vi "Build Tx-UDP Cluster.vi"(0 "section ref in":T8=18446744073709551615 format="%.0x", 5 "board properties":T4 {"portConfig" items=["FDX_SINGLE", "FDX_REDUNDANT"]; "portSpeed" items=["FDX_100MBIT", "FDX_10MBIT", "FDX_AUTO_100MBIT", "FDX_AUTO_10MBIT", "FDX_AUTO_ERROR", "FDX_1000MBIT"]}, 9 "port properties":T3, 11 "error in":errorcluster) -> (4 "section ref out":T8 format="%.0x", 6 "boardId":u32, 8 "portId":u32, 10 "VL Configurations":T7(array[cluster]) {"VL Config"."NetSelect" items=["FDX_TX_FRAME_DLY_A"=0, "FDX_TX_FRAME_DLY_B"=1, "FDX_TX_FRAME_BOTH "=3, "FDX_TX_FRAME_ONLY_A"=4, "FDX_TX_FRAME_ONLY_B "=5]; "VL Config"."interfaceID" format="%.0b"}, 14 "CommPort Payload":T2(array[cluster]), 15 "error out":errorcluster)   [LabVIEW 2020, in "AIM ARINC 664 Scripting.lvlib"]
uses:
  AIM ARINC 664 Scripting.lvlib
  <vilib>/NI VeriStand/Custom Device API/Custom Device Item Ref.ctl
  <instrlib>/AIM GmbH/_AIM 664/_controls/comm_config_vl_tx.ctl
  <instrlib>/AIM GmbH/_AIM 664/_controls/comm_udp_tx.ctl
  Shared/board_setup.ctl
  Shared/port_setup.ctl
  <vilib>/NI/NI VeriStand Encoding and Decoding/Encoding.ctl
  <instrlib>/AIM GmbH/_AIM 664/AIM664LV.lvlib
  <vilib>/NI VeriStand/Custom Device API/Custom Device API.lvlib
  <vilib>/NI/NI VeriStand Encoding and Decoding/Encoding and Decoding.lvlib
  Import/AIM ARINC 664 Import.lvlib
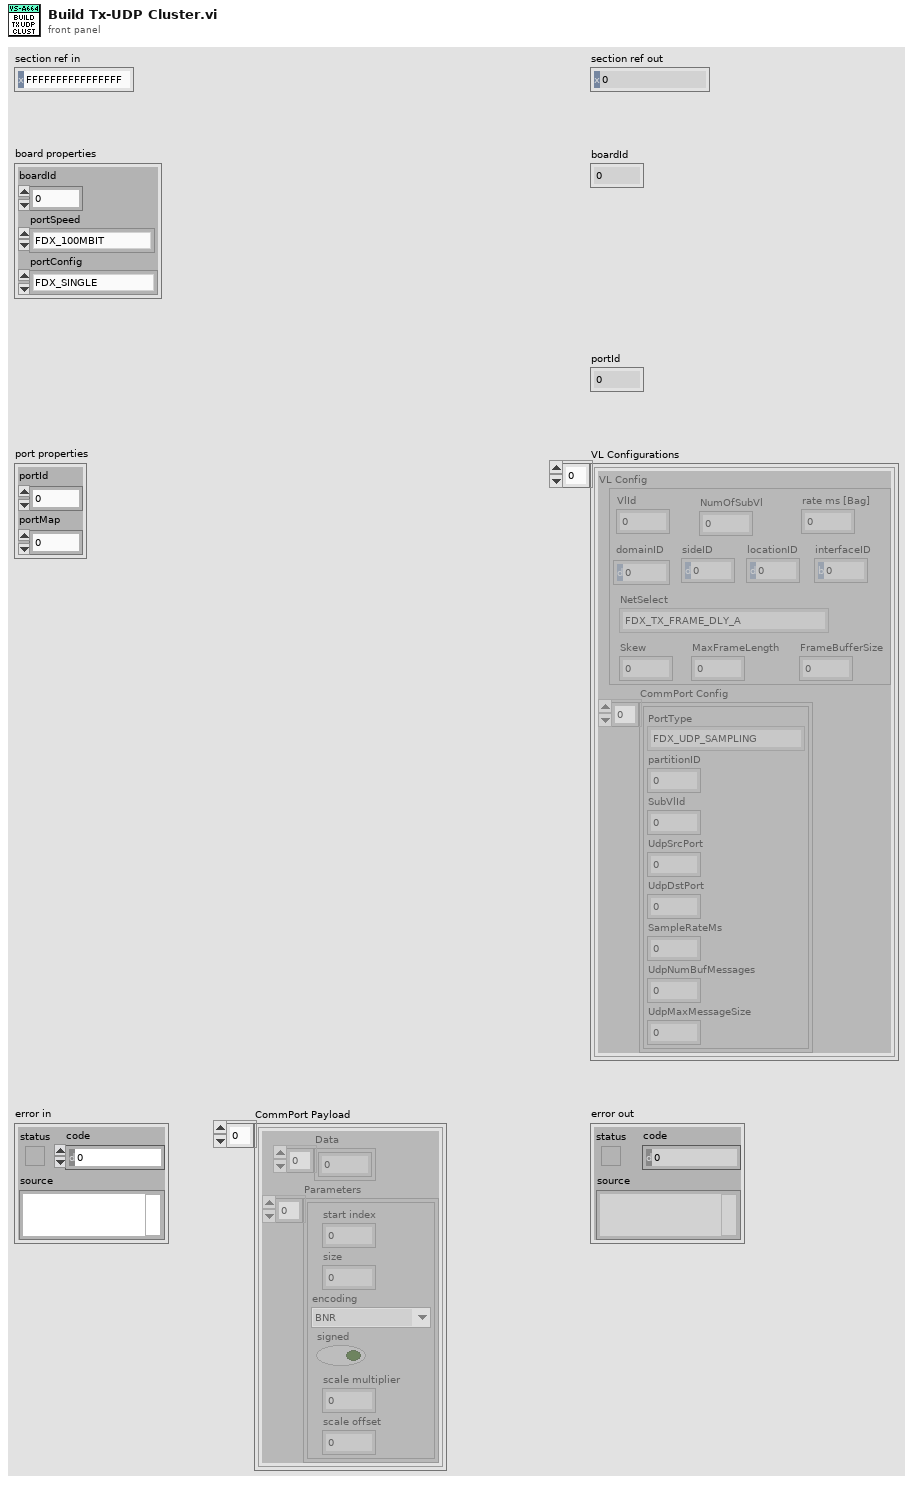
[diagram p1: front panel]
types:
  T1 = typedef "Encoding and Decoding.lvlib/Encoding.ctl" = enum16{"BNR", "BCD", "Discrete"}
  T2 = cluster{"Data":u8[], "Parameters":cluster{"start index":i32, "size":i32, "encoding":T1, "signed":bool, "scale multiplier":dbl, "scale offset":dbl}[]}[]
  T3 = typedef "AIM ARINC 664 Import.lvlib/port_setup.ctl" = cluster{"portId":u32, "portMap":u32}
  T4 = typedef "AIM ARINC 664 Import.lvlib/board_setup.ctl" = cluster{"boardId":u32, "portSpeed":u32, "portConfig":u32}
  T5 = typedef "AIM664LV.lvlib/comm_config_vl_tx.ctl" = cluster{"VlId":u16, "NumOfSubVl":u16, "rate ms [Bag]":u32, "domainID":u8, "sideID":u8, "locationID":u8, "interfaceID":u8, "NetSelect":u32, "Skew":u32, "MaxFrameLength":u32, "FrameBufferSize":u32}
  T6 = typedef "AIM664LV.lvlib/comm_udp_tx.ctl" = cluster{"PortType":enum16{"FDX_UDP_SAMPLING", "FDX_UDP_QUEUING"}, "partitionID":u8, "SubVlId":u8, "UdpSrcPort":u16, "UdpDstPort":u16, "SampleRateMs":dbl, "UdpNumBufMessages":u32, "UdpMaxMessageSize":u32}
  T7 = cluster{"VL Config":T5, "CommPort Config":T6[]}[]
  T8 = typedef "Custom Device API.lvlib/Custom Device Item Ref.ctl" = u64
  T9 = cluster{"Data":u8[], "Parameters":cluster{"start index":i32, "size":i32, "encoding":T1, "signed":bool, "scale multiplier":dbl, "scale offset":dbl}[]}
  T10 = cluster{"start index":i32, "size":i32, "encoding":T1, "signed":bool, "scale multiplier":dbl, "scale offset":dbl}
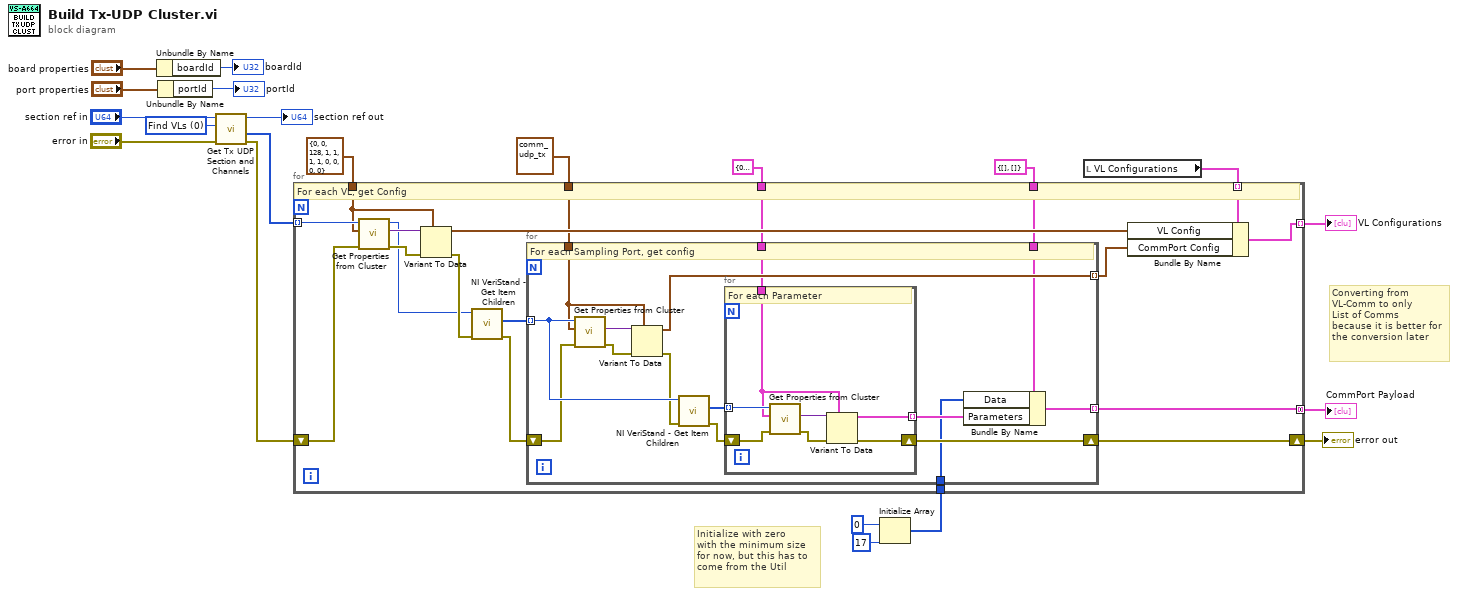
[diagram p0: block diagram]
diagram:
  w16 = u16 0 items=["Find VLs", "Find Parameters"] ("Option")
  # "Initialize with zero\nwith the minimum size\nfor now, but this has to\ncome from the Util"
  # "Converting from \nVL-Comm to only\nList of Comms\nbecause it is better for\nthe conversion later"
  n1 = Unbundle By Name("board properties") -> ("boardId"=→"boardId":u32)
  n2 = Unbundle By Name("port properties") -> ("portId"=→"portId":u32)
  n3 = call "Get Tx UDP Section and Channels.vi"("error in"="error in", "Option"=w16, "Custom Device Ref in"="section ref in") -> ("error out"=w12:errorcluster, "Channel Refs Out"=w11:T8[], "Custom Device Ref out"=→"section ref out":T8)  [unwired: 4 in, 2 out]
  n4 = Initialize Array(u8 0 ("Numeric"), 17 ("dimension size")) -> (w1:u8[])
  n5 = local read "VL Configurations"() -> (w9:T7)
  n6 = for {
    tunnel: [w29] -> w19 mode=indexing
    tunnel: w11 -> [w40] mode=indexing
    tunnel: T5 {"VlId"=0, "NumOfSubVl"=0, "rate ms [Bag]"=128, "domainID"=1, "sideID"=1, "locationID"=1, "interfaceID"=1, "NetSelect"=0, "Skew"=0, "MaxFrameLength"=0, "FrameBufferSize"=0} ("CommPort Config") -> [w38]
    shift-right: [w23] -> w4
    shift-left: w12 -> [w39]
    tunnel: w9 -> [w31] mode=indexing
    tunnel: T6 {"PortType"=enum."FDX_UDP_SAMPLING", "partitionID"=0, "SubVlId"=1, "UdpSrcPort"=0, "UdpDstPort"=0, "SampleRateMs"=128.0, "UdpNumBufMessages"=0, "UdpMaxMessageSize"=0} ("commPort config") -> [w28]
    tunnel: T10 {"start index"=0, "size"=0, "encoding"=enum."BNR", "signed"=FALSE, "scale multiplier"=0.0, "scale offset"=0.0} ("Parameter") -> [w26]
    tunnel: [w24] -> w6 mode=concatenating
    tunnel: T9 {"Data"=[], "Parameters"=[]} ("Data and Parameters") -> [w25]
    tunnel: w1 -> [w22]
    # "For each VL, get Config"
    n7 = call "Get Properties from Cluster.vi"("error in"=w39, "Variant Cluster"=w38, "custom device ref in"=w40) -> ("error out"=w36:errorcluster, "data"=w37:variant, "custom device ref out"=w34:T8)  [unwired: 5 in, 1 out]
    n8 = Variant To Data(error in=w36, type=w38, Variant=w37) -> (data=w30:T5, error out=w35:errorcluster)
    n9 = call <vilib>:"NI VeriStand - Get Item Children.vi"("error in (no error)"=w35, "Item Ref in"=w34) -> ("error out"=w32:errorcluster, "Child Refs"=w33:T8[])  [unwired: 6 in, 2 out]
    n10 = for {
      tunnel: w33 -> [w51] mode=indexing
      shift-right: [w44] -> w23
      shift-left: w32 -> [w43]
      tunnel: w28 -> [w50]
      tunnel: [w49] -> w27 mode=indexing
      tunnel: w26 -> [w48]
      tunnel: w25 -> [w47]
      tunnel: [w45] -> w24 mode=indexing
      tunnel: w22 -> [w41]
      # "For each Sampling Port, get config"
      n11 = call "Get Properties from Cluster.vi"("error in"=w43, "Variant Cluster"=w50, "custom device ref in"=w51) -> ("error out"=w53:errorcluster, "data"=w52:variant)  [unwired: 5 in, 2 out]
      n12 = Variant To Data(error in=w53, type=w50, Variant=w52) -> (data=w49:T6, error out=w42:errorcluster)
      n13 = call <vilib>:"NI VeriStand - Get Item Children.vi"("error in (no error)"=w42, "Item Ref in"=w51) -> ("error out"=w54:errorcluster, "Child Refs"=w55:T8[])  [unwired: 6 in, 2 out]
      n14 = for {
        tunnel: w55 -> [w60] mode=indexing
        shift-right: [w56] -> w44
        shift-left: w54 -> [w57]
        tunnel: w48 -> [w59]
        tunnel: [w58] -> w46 mode=indexing
        # "For each Parameter"
        n15 = call "Get Properties from Cluster.vi"("error in"=w57, "Variant Cluster"=w59, "custom device ref in"=w60) -> ("error out"=w61:errorcluster, "data"=w62:variant)  [unwired: 5 in, 2 out]
        n16 = Variant To Data(error in=w61, type=w59, Variant=w62) -> (data=w58:T10, error out=w56:errorcluster)
      }
      n17 = Bundle By Name(cluster=w47, "Data"=w41, "Parameters"=w46) -> (w45:T9)
    }
    n18 = Bundle By Name(cluster=w31, "VL Config"=w30, "CommPort Config"=w27) -> (w29:cluster{"VL Config":T5, "CommPort Config":T6[]})
  }
  "error out" <- w4
  "VL Configurations" <- w19
  "CommPort Payload" <- w6
